vi "resetView.vi"(8 "error in (no error)":errorcluster, 11 "BankingListUserInterface in":refnum<class "BankingListUserInterface.lvclass">) -> (0 "error out":errorcluster, 3 "BankingListUserInterface out":refnum<class "BankingListUserInterface.lvclass">)   [LabVIEW 2018, in "BankingListUserInterface.lvclass"]
uses:
  BankingListUserInterface.lvclass
  TransactionListUserInterface/TransactionListUserInterface.lvclass
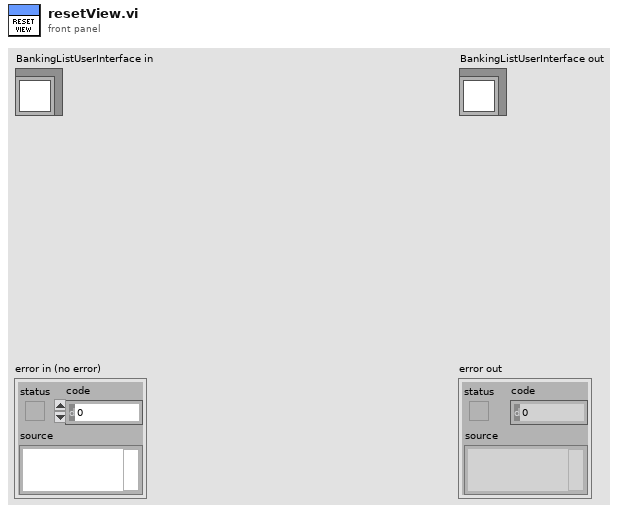
[diagram p1: front panel]
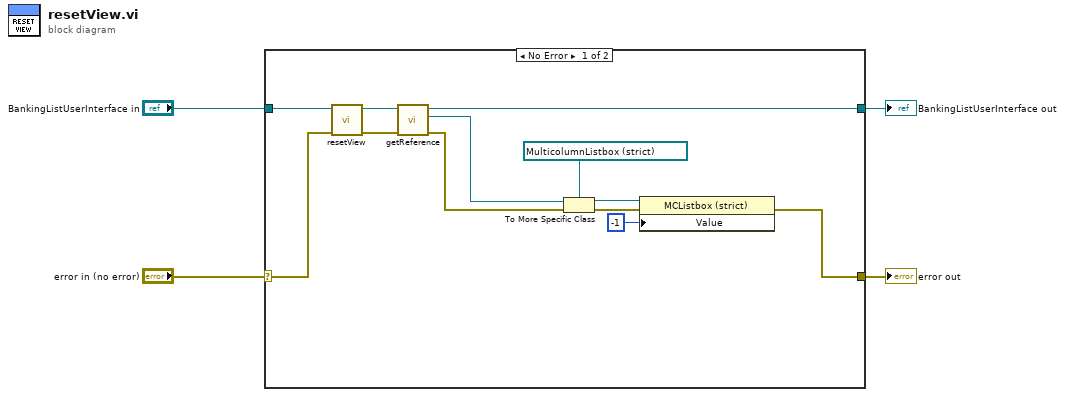
[diagram p0: block diagram]
diagram:
  n1 = case shown="No Error" "error in (no error)" {
    selector: "error in (no error)" -> [w14 w18]
    tunnel: [w16 w18] -> w3
    tunnel: [w10 w17] -> w1
    tunnel: "BankingListUserInterface in" -> [w15 w17]
    frame No Error {
      n2 = call-parent "resetView.vi"("error in (no error)"=w14, "TransactionListUserInterface in"=w15) -> ("error out"=w11:errorcluster, "TransactionListUserInterface out"=w12:refnum<class "BankingListUserInterface.lvclass">)  [unwired: 8 in]
      n3 = call-dynamic "getReference.vi"("error in (no error)"=w11, "TransactionListUserInterface in"=w12) -> ("error out"=w8:errorcluster, "MulticolumnListbox"=w9:refnum<vi>, "TransactionListUserInterface out"=w10:refnum<class "BankingListUserInterface.lvclass">)  [unwired: 7 in]
      n4 = To More Specific Class(target class=refnum<vi> refnum ("Banking"), reference=w9, error in=w8) -> (specific class reference=w6:refnum<vi>, error out=w7:errorcluster)
      n5 = property on="Property Node" class="MCListbox (strict)"(reference=w6, error in=w7, "Value"=-1 ("Banking")) -> (error out=w16:errorcluster)  [unwired: 1 out]
    }
    frame Error {
    }
  }
  "error out" <- w3
  "BankingListUserInterface out" <- w1
